vi "Page_Info_Write.vi"(6 "ctlReferences":T1, 8 "error in (no error)":errorcluster, 10 "Target filename":string, 11 "AB_Targetfile in":refnum<class "AB_Targetfile.lvclass">) -> (0 "error out":errorcluster, 3 "AB_Targetfile out":refnum<class "AB_Targetfile.lvclass">)   [LabVIEW 2020, in "AB_Targetfile.lvclass"]
uses:
  <vilib>/AppBuilder/AB_Classes/TargetFile/AB_Targetfile.lvclass
  e:/builds/penguin/labview/branches/2020/dev/dist/vi.lib/AppBuilder/AB_Classes/Build/AB_Build.lvclass
  <resource>/Framework/Providers/Builds/AppBuilder/AB_UI_Page_Info_References.ctl
  <vilib>/AppBuilder/AB_Classes/Build/AB_Build.lvclass
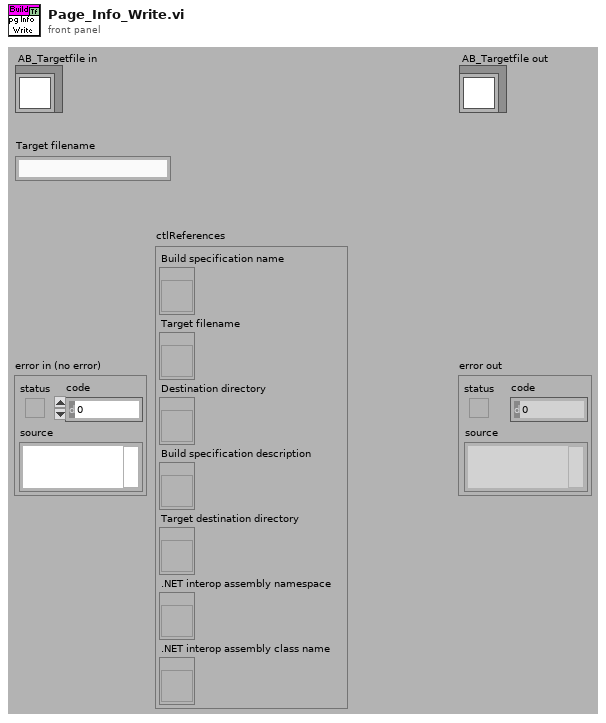
[diagram p1: front panel]
types:
  T1 = typedef "AB_UI_Page_Info_References.ctl" = cluster{"Build specification name":refnum<vi>, "Target filename":refnum<vi>, "Destination directory":refnum<vi>, "Build specification description":refnum<vi>, "Target destination directory":refnum<vi>, ".NET interop assembly namespace":refnum<vi>, ".NET interop assembly class name":refnum<vi>}
  T2 = typedef "AB_Build.ctl" = cluster{"buildSpecName":string, "buildSpecDescription":string, "destinations":refnum<class "AB_Destination.lvclass">[], "exclusionOption":T3, "defaultLanguage":string, "supportedLanguages":string[], "excludedDirectories":path[], "buildContext":refnum<vi>, "buildObject":T4, "preview":bool, "programatic":bool, "progressBarEvents":T5, "userLog_Path":path, "preActionID":string, "preAction_Path":path, "postActionID":string, "postAction_Path":path, "eng_checkForBrokenVIs?":bool, "eng_verboseLinkerErrors?":bool, "localDest_Path":path, "targetDest_Path":path, "removeVIObject":u16, "cache":refnum<class "PreviewCache.lvclass">, "use cache":bool, "previewCache_ID":string, "buildCache_ID":string, "eng_TempLocalDest_Path":path, "eng_collectDependencies?":bool, "versionInfo":cluster{"buildVersion":cluster{"major":u16, "minor":u16, "patch":u16, "build":u16}, "autoIncrement":bool}, "eng_enableVIChecksums":bool}
  T3 = typedef "AB_Exclusion_Option.ctl" = cluster{"typedefs":bool, "polymorphicVIs":bool, "unusedLibraryItems":bool, "modifyLibraryFile":bool, "edit-timeDependencies":bool, "inlineVIs":bool, "dependent PPLs":bool, "dependent DLLs":bool}
  T4 = typedef "ItemRef.ctl" = u64
  T5 = typedef "provcom_ProgressBar_Events.ctl" = cluster{"newJob":refnum<user-event>, "newItem":refnum<user-event>, "errorMsg":T6, "cancel":refnum<user-event>}
  T6 = typedef "mxLvBuildError.ctl" = refnum<user-event>
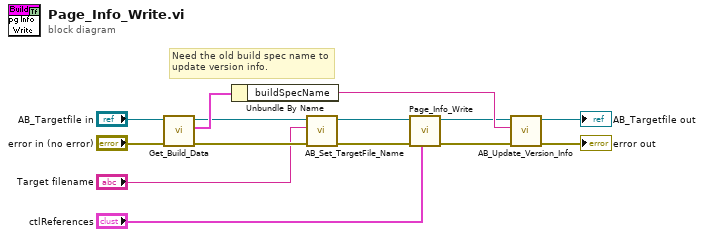
[diagram p0: block diagram]
diagram:
  # "Need the old build spec name to update version info."
  n1 = call <vilib>:"Get_Build_Data.vi"("error in (no error)"="error in (no error)", "Class in"="AB_Targetfile in") -> ("error out"=w9:errorcluster, "data"=w13:T2, "Class out"=w12:refnum<class "AB_Targetfile.lvclass">)  [unwired: 7 in]
  n2 = Unbundle By Name(w13) -> ("buildSpecName"=w5:string)
  n3 = call <vilib>:"AB_Set_TargetFile_Name.vi"("error in (no error)"=w9, "Target filename"="Target filename", "TargetFile in"=w12) -> ("error out"=w11:errorcluster, "TargetFile out"=w2:refnum<class "AB_Targetfile.lvclass">)  [unwired: 7 in]
  n4 = call-parent "Page_Info_Write.vi"("ctlReferences"="ctlReferences", "error in (no error)"=w11, "AB_Build in"=w2) -> ("error out"=w6:errorcluster, "AB_Build out"=w4:refnum<class "AB_Targetfile.lvclass">)  [unwired: 7 in]
  n5 = call <vilib>:"AB_Update_Version_Info.vi"("error in (no error)"=w6, "Build spec name"=w5, "TargetFile in"=w4) -> ("error out"=→"error out":errorcluster, "TargetFile out"=→"AB_Targetfile out":refnum<class "AB_Targetfile.lvclass">)  [unwired: 7 in]
